vi "Init Package Version.vi"(6 "Product Name":string, 7 "Dev Mode":bool, 8 "error in":errorcluster) -> (0 "error out":errorcluster, 3 "VIP Package Version":string)   [LabVIEW 2014, in "Raspberry Pi Compatible Compiler for LabVIEW.lvlib"]
uses:
  Raspberry Pi Compatible Compiler for LabVIEW.lvlib
  RasPi_Services/Download/RuntimeVersion.ctl
  Compile and Download App/Custom Controls/Local Setup Parameters.ctl
  RasPi_Services/Download/RasPiDownloader.lvlib
panel:
  out "Version":T1
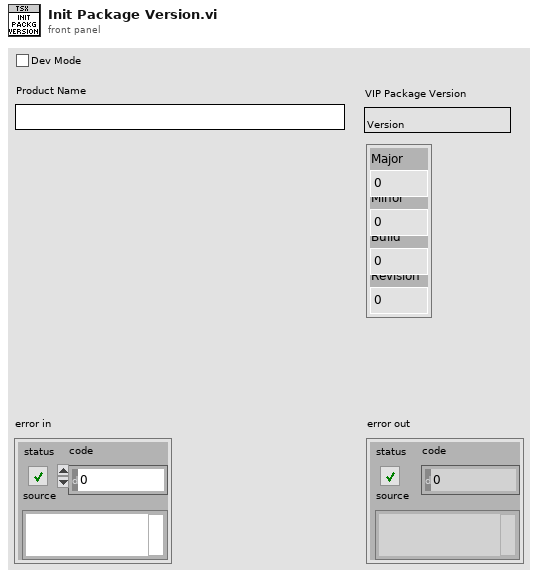
[diagram p1: front panel]
types:
  T1 = typedef "Raspberry Pi Compatible Compiler for LabVIEW.lvlib/RasPiDownloader.lvlib/RuntimeVersion.ctl" = cluster{"Major":i32, "Minor":i32, "Build":i32, "Revision":i32}
  T2 = typedef "Raspberry Pi Compatible Compiler for LabVIEW.lvlib/Local Setup Parameters.ctl" = enum16{"Add Last VI", "Read Last VI", "Add Board IP", "Remove Board IP", "Read All Board IP", "Add Runtime Version", "Read Runtime Version", "Add Package Version", "Read Package Version", "Add VIPCheck Time", "Read VIPCheck Time"}
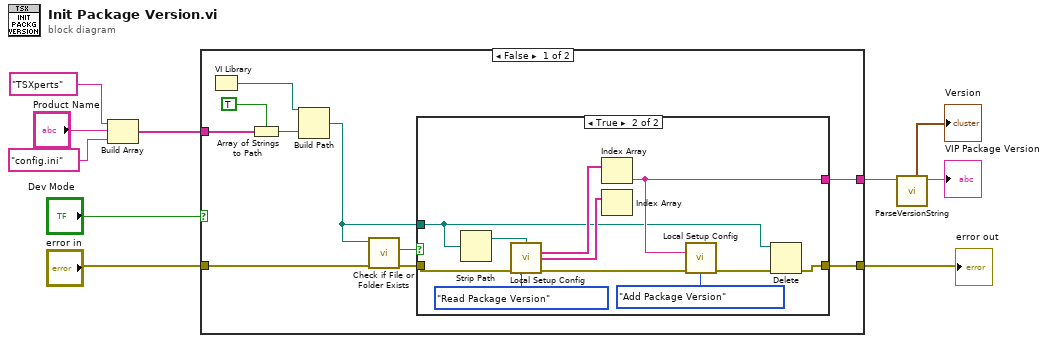
[diagram p0: block diagram]
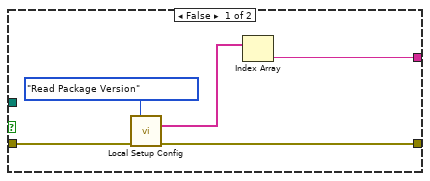
[diagram p2: hidden frame]
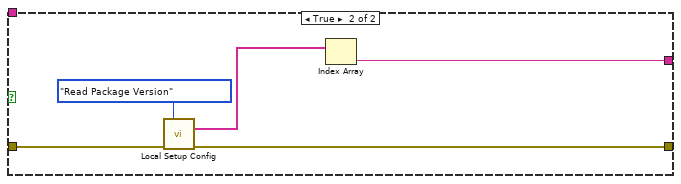
[diagram p3: hidden frame]
diagram:
  n1 = Build Array("TSXperts" ("name or relative path"), "Product Name", "config.ini" ("string")) -> (w5:string[])
  n2 = case shown="False" "Dev Mode" {
    tunnel: "error in" -> [w19 w41]
    tunnel: [w16 w40] -> w9
    tunnel: [w15 w37] -> w2
    tunnel: w5 -> [w20 _]
    frame False {
      n3 = VI Library() -> (path=w13:path)
      n4 = Array of Strings to Path(0:w20, 1:TRUE ("relative")) -> (2:w12:path)
      n5 = Build Path(base path=w13, name or relative path=w12) -> (appended path=w14:path)
      n6 = call <vilib>:"Check if File or Folder Exists.vi"("error in (no error)"=w19, "path"=w14) -> ("error out"=w17:errorcluster, "file or folder exists?"=w18:bool)  [unwired: 7 in, 1 out]
      n7 = case shown="True" w18 {
        tunnel: w17 -> [w23 w34]
        tunnel: [w22 w32] -> w16
        tunnel: [w21 w31] -> w15
        tunnel: w14 -> [_ w26]
        frame False {
          n8 = call "Local Setup Config.vi"("Local Setup Param"=Local_Setup_Parameters."Read Package Version", "error in"=w23) -> ("KeyValues"=w24:string[], "error out"=w22:errorcluster)  [unwired: 10 in, 2 out]
          n9 = Index Array(array=w24) -> (element=w21:string)  [unwired: 1 in]
        }
        frame True {
          n10 = Strip Path(path=w26) -> (stripped path=w27:path)  [unwired: 1 out]
          n11 = call "Local Setup Config.vi"("Local Setup Param"=Local_Setup_Parameters."Read Package Version", "Config File Directory"=w27, "error in"=w34) -> ("KeyValues"=w35:string[], "KeyNames"=w33:string[], "error out"=w30:errorcluster)  [unwired: 9 in, 1 out]
          n12 = Index Array(array=w35) -> (element=w31:string)  [unwired: 1 in]
          n13 = Index Array(array=w33) -> ()  [unwired: 1 in, 1 out]
          n14 = call "Local Setup Config.vi"("Local Setup Param"=Local_Setup_Parameters."Add Package Version", "KeyValue"=w31, "error in"=w30) -> ("error out"=w28:errorcluster)  [unwired: 9 in, 3 out]
          n15 = Delete(path (use dialog)=w26, error in=w28) -> (error out=w32:errorcluster)  [unwired: 3 in, 2 out]
        }
      }
    }
    frame True {
      n16 = call "Local Setup Config.vi"("Local Setup Param"=Local_Setup_Parameters."Read Package Version", "error in"=w41) -> ("KeyValues"=w38:string[], "error out"=w40:errorcluster)  [unwired: 10 in, 2 out]
      n17 = Index Array(array=w38) -> (element=w37:string)  [unwired: 1 in]
    }
  }
  "error out" <- w9
  n18 = call "ParseVersionString.vi"("version string"=w2) -> ("fixed version string"=→"VIP Package Version":string, "Version"=→"Version":T1)  [unwired: 7 in]
